vi "ObtainNotifiers.vi"(11 "create if not found? (F)":bool) -> (2 "SettingsActuators":refnum<notifier>, 3 "Sensors":refnum<notifier>)   [LabVIEW 2019]
uses:
  Sensors_State.ctl
  Settings_Actuators.ctl
panel:
  out "error out":errorcluster
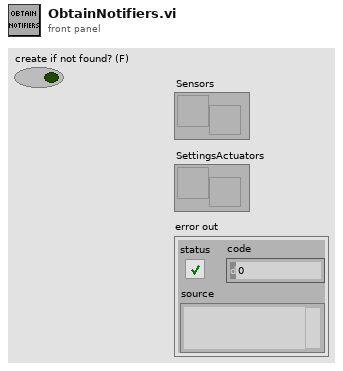
[diagram p1: front panel]
types:
  T1 = typedef "Sensors_State.ctl" = cluster{"Kiuas_Button":bool, "Loyly_Button":bool, "Aromi_Button":bool, "Door":bool, "Ceiling_Temp":dbl, "Kiuas_Temp":dbl, "Aromi_Volume":dbl}
  T2 = typedef "Settings_Actuators.ctl" = cluster{"Kiuas_Button_LED":bool, "Loyly_Button_LED":bool, "Loyly_Valve_Enable":bool, "Loyly_Valve":bool, "Aromi_Button_LED":bool, "Aromi_Pump_Enable":bool, "Aromi_Pump":bool, "Aromi_Pump_Direction":bool, "Aromi_Pump_Cycle":u32}
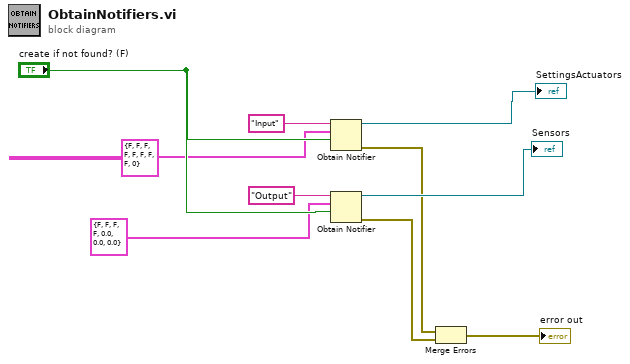
[diagram p0: block diagram]
diagram:
  n1 = Obtain Notifier(name (unnamed)="Input", notification data type=T2 {"Kiuas_Button_LED"=FALSE, "Loyly_Button_LED"=FALSE, "Loyly_Valve_Enable"=FALSE, "Loyly_Valve"=FALSE, "Aromi_Button_LED"=FALSE, "Aromi_Pump_Enable"=FALSE, "Aromi_Pump"=FALSE, "Aromi_Pump_Direction"=FALSE, "Aromi_Pump_Cycle"=0} ("SettingsActuators"), create if not found? (T)="create if not found? (F)") -> (notifier out=→"SettingsActuators":refnum<notifier>, error out=w6:errorcluster)  [unwired: 1 in, 1 out]
  n2 = Obtain Notifier(name (unnamed)="Output", notification data type=T1 {"Kiuas_Button"=FALSE, "Loyly_Button"=FALSE, "Aromi_Button"=FALSE, "Door"=FALSE, "Ceiling_Temp"=0.0, "Kiuas_Temp"=0.0, "Aromi_Volume"=0.0} ("SensorsState"), create if not found? (T)="create if not found? (F)") -> (notifier out=→"Sensors":refnum<notifier>, error out=w7:errorcluster)  [unwired: 1 in, 1 out]
  n3 = Merge Errors(w6, w7) -> (→"error out":errorcluster)
